vi "Test BOOL Write_Read.vi"(8 "error in (no error)":errorcluster, 11 "Scalar Channels Testing in":refnum<class "Scalar Channels Testing.lvclass">) -> (0 "error out":errorcluster, 3 "Scalar Channels Testing out":refnum<class "Scalar Channels Testing.lvclass">)   [LabVIEW 2019, in "Scalar Channels Testing.lvclass"]
uses:
  Scalar Channels Testing.lvclass
  C:/Program Files (x86)/National Instruments/LabVIEW 2019/vi.lib/NI/NI VeriStand Development Tools/NI Veristand Test Utilities/VeriStandTestCase/VeriStandTestCase.lvclass
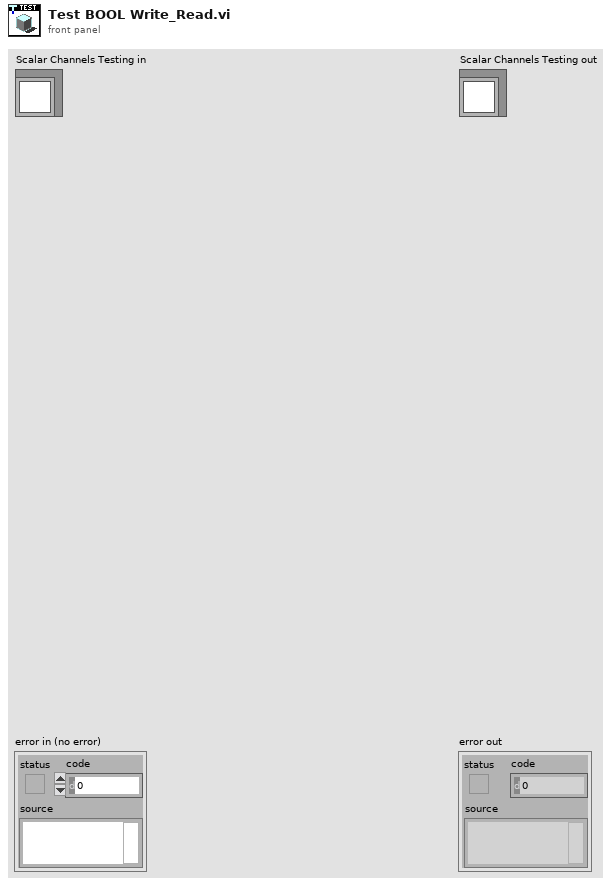
[diagram p1: front panel]
types:
  T1 = typedef "NI_VS Workspace ExecutionAPI.lvlib/WorkspaceAPI.ctl" = refnum<k24>
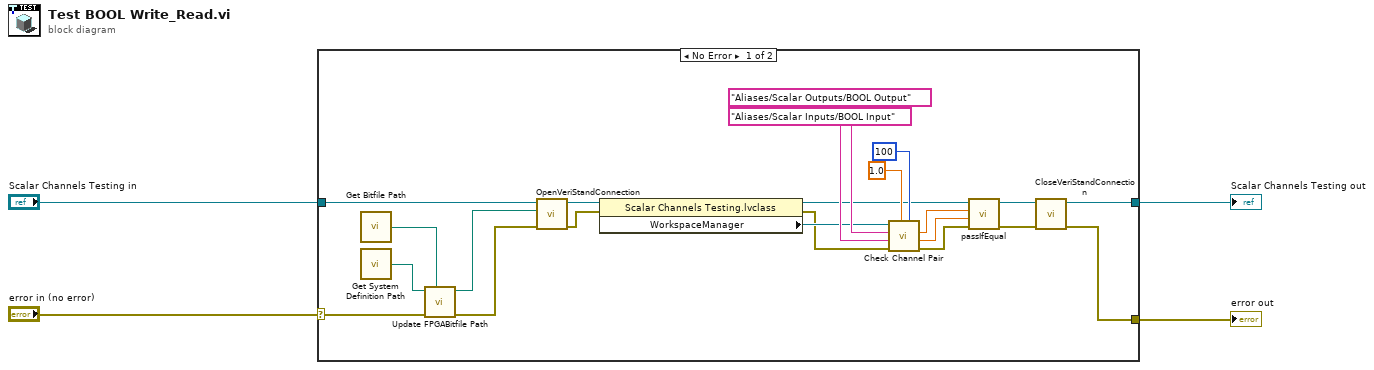
[diagram p0: block diagram]
diagram:
  n1 = case shown="No Error" "error in (no error)" {
    selector: "error in (no error)" -> [w7 w28]
    tunnel: [w24 w28] -> w3
    tunnel: [w25 w27] -> w1
    tunnel: "Scalar Channels Testing in" -> [w26 w27]
    frame No Error {
      n2 = call "Get Bitfile Path.vi"() -> ("Bitfile Path"=w8:path)
      n3 = call "Get System Definition Path.vi"() -> ("System Definition path"=w9:path)
      n4 = call "Update FPGABitfile Path.vi"("Bitfile Path"=w8, "error in (no error)"=w7, "System Definition path in"=w9) -> ("error out"=w6:errorcluster, "System Definition path out"=w5:path)  [unwired: 7 in]
      n5 = call-dynamic "OpenVeriStandConnection.vi"("error in (no error)"=w6, "System Definition File"=w5, "VeriStand Test Case in"=w26) -> ("error out"=w19:errorcluster, "VeriStand Test Case out"=w18:refnum<class "Scalar Channels Testing.lvclass">)  [unwired: 6 in, 1 out]
      n6 = property class="Scalar Channels Testing.lvclass"(reference=w18, error in=w19) -> (reference out=w15:refnum<class "Scalar Channels Testing.lvclass">, error out=w16:errorcluster, "WorkspaceManager"=w17:T1)
      n7 = call "Check Channel Pair.vi"("milliseconds to wait"=u32 100, "Test Value"=1.0 ("Value"), "error in (no error)"=w16, "Input Channel"="Aliases/Scalar Inputs/BOOL Input" ("Channel"), "Output Channel"="Aliases/Scalar Outputs/BOOL Output" ("Channel"), "WorkspaceManager in"=w17) -> ("error out"=w11:errorcluster, "InputChannel Value"=w13:dbl, "OutputChannel Value"=w14:dbl)  [unwired: 2 in, 1 out]
      n8 = call-dynamic "passIfEqual.vi"("error in (no error)"=w11, "y"=w13, "x"=w14, "TestCase in"=w15) -> ("error out"=w10:errorcluster, "TestCase out"=w12:refnum<class "Scalar Channels Testing.lvclass">)  [unwired: 6 in]
      n9 = call-dynamic "CloseVeriStandConnection.vi"("error in (no error)"=w10, "VeriStand Test Case in"=w12) -> ("error out"=w24:errorcluster, "VeriStand Test Case out"=w25:refnum<class "Scalar Channels Testing.lvclass">)  [unwired: 8 in]
    }
    frame Error {
    }
  }
  "error out" <- w3
  "Scalar Channels Testing out" <- w1
